vi "test_sicm_main2.vi"() -> ()   [LabVIEW 2016]
uses:
  <vilib>/rvi/DesktopExecutionNode/Execution/niFpgaDEN_Execute.vi
  <vilib>/rvi/DesktopExecutionNode/DesktopExecutionNode.xnode
panel:
  out "Baseline":dbl[](graph)
  out "Height":dbl[](graph)
  out "current":dbl[](graph)
  out "Baseline":T1(array[cluster])
  out "Debug":T2(array[cluster])
  out "Trigger":T3(array[cluster])
  in  "sicm.p.modes":T4
  in  "sicm.display":cluster{"sicm.ptsAfterTrig":u16}={"sicm.ptsAfterTrig"=10}
  in  "sicm.p.params":T5={"sicm.p.setPoint"=0.9700002670288086, "sicm.p.setPointFrac"=-33.328125, "stepDown"=0.001999974250793457, "retractHeight"=-0.19999998807907104, "adaptiveMin"=0.099609375}
  out "heightOut":T6(array[cluster])
  in  "enablethicks":i32=2000
  out "Progress":dbl(slide)=0.9999 scale=0.0..1.0
  in  "sicm.i.current":T7
  in  "sicm.p.clocks":T8={"inverseDecimation"=0.03332996368408203, "decimation"=10, "waveSize"=128, "pixelDecimation"=0}
  in  "sicm.blc.p.params":T9={"se.blc.p.postRetractDelay"=1000, "se.blc.p.windowSize"=20, "se.blc.p.updateFactor"=-5, "blc.resetBackground"=FALSE}
  in  "d0":dbl=0.3
  in  "D":dbl=0.05
  in  "Idc":dbl=5000.0
  in  "Simulation ticks":i32=10000
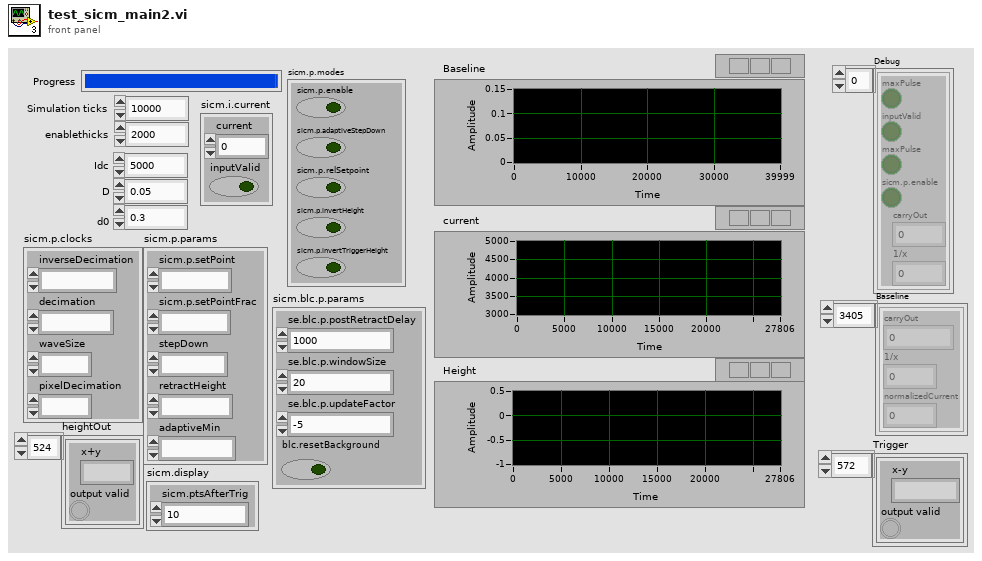
[diagram p1: front panel]
types:
  T1 = cluster{"carryOut":fxp<+/-,22,2>, "1/x":fxp<+/-,32,24>, "normalizedCurrent":fxp<+,20,1>}[]
  T2 = cluster{"maxPulse":bool, "inputValid":bool, "maxPulse":bool, "sicm.p.enable":bool, "carryOut":fxp<+/-,22,2>, "1/x":fxp<+/-,27,24>}[]
  T3 = cluster{"x-y":fxp<+/-,22,4>, "output valid":bool}[]
  T4 = cluster{"sicm.p.enable":bool, "sicm.p.adaptiveStepDown":bool, "sicm.p.relSetpoint":bool, "sicm.p.invertHeight":bool, "sicm.p.invertTriggerHeight":bool}
  T5 = cluster{"sicm.p.setPoint":fxp<+,20,0>, "sicm.p.setPointFrac":fxp<+/-,20,14>, "stepDown":fxp<+/-,28,4>, "retractHeight":fxp<+/-,28,4>, "adaptiveMin":fxp<+,10,0>}
  T6 = cluster{"x+y":fxp<+/-,28,2>, "output valid":bool}[]
  T7 = cluster{"current":fxp<+/-,24,16>, "inputValid":bool}
  T8 = cluster{"inverseDecimation":fxp<+,22,0>, "decimation":u16, "waveSize":u16, "pixelDecimation":u16}
  T9 = cluster{"se.blc.p.postRetractDelay":u16, "se.blc.p.windowSize":u16, "se.blc.p.updateFactor":i16, "blc.resetBackground":bool}
  T10 = cluster{"x-y":fxp<+/-,22,4>, "output valid":bool}
  T11 = cluster{"x+y":fxp<+/-,28,2>, "output valid":bool}
  T12 = cluster{"maxPulse":bool, "inputValid":bool, "maxPulse":bool, "sicm.p.enable":bool, "carryOut":fxp<+/-,22,2>, "1/x":fxp<+/-,27,24>}
  T13 = cluster{"carryOut":fxp<+/-,22,2>, "1/x":fxp<+/-,32,24>, "normalizedCurrent":fxp<+,20,1>}
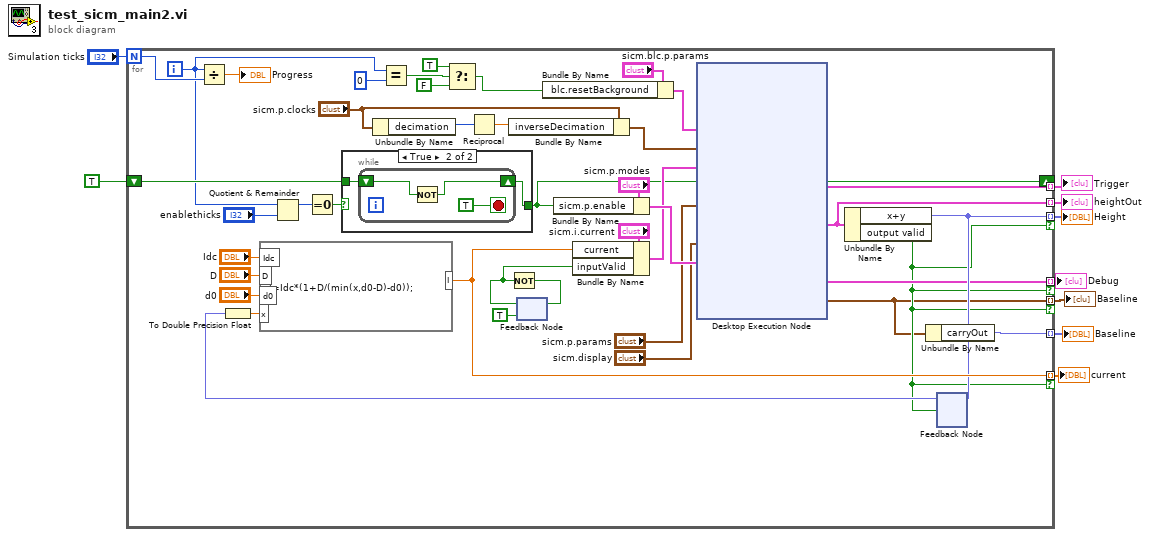
[diagram p0: block diagram]
diagram:
  n1 = for {
    N: "Simulation ticks" -> [w48]
    tunnel: [w35] -> w8 mode=indexing if=w21
    tunnel: [w34] -> w7 mode=indexing
    tunnel: [w31] -> w6 mode=indexing
    tunnel: [w28] -> w5 mode=indexing if=w21
    shift-right: [w20] -> _
    shift-left: TRUE -> [w23]
    tunnel: [w22] -> w3 mode=indexing if=w21
    tunnel: [w19] -> w2 mode=indexing if=w21
    tunnel: [w18] -> w1 mode=indexing
    i -> [w15]
    n2 = Divide(x=w15, y=w48) -> (x/y=→"Progress":dbl)
    n3 = Quotient & Remainder(x=w15, y="enablethicks") -> (x-y*floor(x/y)=w25:i32)  [unwired: 1 out]
    n4 = Equal To 0?(x=w25) -> (x = 0?=w24:bool)
    n5 = case shown="True" w24 {
      tunnel: w23 -> [w51 w53]
      tunnel: [w51 w52] -> w20
      frame False {
      }
      frame True {
        n6 = while {
          shift-right: [w55] -> w52
          shift-left: w53 -> [w54]
          stop <- TRUE stop-if-true
          n7 = Not(x=w54) -> (.not. x?=w55:bool)
        }
      }
    }
    n8 = Unbundle By Name("sicm.p.clocks") -> ("decimation"=w36:u16)
    n9 = Equal?(x=w15, y=0) -> (x = y?=w12:bool)
    n10 = Select(t=TRUE, s=w12, f=FALSE) -> (s? t:f=w13:bool)
    n11 = Reciprocal(x=w36) -> (1/x=w37:dbl)
    n12 = Bundle By Name(cluster="sicm.p.clocks", "inverseDecimation"=w37) -> (w39:T8)
    n13 = feedback #1(TRUE) -> (w40:bool)
    n14 = Not(x=w40) -> (.not. x?=w42:bool)
    n15 = feedback-in #1(w42) -> ()
    n16 = Bundle By Name(cluster="sicm.blc.p.params", "blc.resetBackground"=w13) -> (w16:T9)
    n17 = Bundle By Name(cluster="sicm.p.modes", "sicm.p.enable"=w20) -> (w50:T4)
    n18 = feedback #2() -> (w30:fxp<+/-,28,2>)  [unwired: 1 in]
    n19 = To Double Precision Float(number=w30) -> (double precision float=w44:dbl)
    n20 = formula code="I=Idc*(1+D/(min(x,d0-D)-d0));"("Idc"="Idc", "D"="D", "d0"="d0", "x"=w44) -> ("I"=w35:dbl)
    n21 = Bundle By Name(cluster="sicm.i.current", "current"=w35, "inputValid"=w40) -> (w43:T7)
    n22 = xnode "Desktop Execution Node"("sicm.blc.p.params"=w16, "sicm.p.clocks"=w39, "sicm.i.current"=w43, "sicm.p.params"="sicm.p.params", "sicm.display"="sicm.display", "sicm.p.modes"=w50) -> ("sicm.triggerHeight"=w34:T10, "heightOut"=w31:T11, "debug"=w22:T12, "sicm.Baseline"=w19:T13)  [unwired: 1 in, 1 out]
    n23 = Unbundle By Name(w31) -> ("x+y"=w28:fxp<+/-,28,2>, "output valid"=w21:bool)
    n24 = Unbundle By Name(w19) -> ("carryOut"=w18:fxp<+/-,22,2>)
    n25 = feedback-in #2(w28, w21) -> ()
  }
  "current" <- w8
  "Trigger" <- w7
  "heightOut" <- w6
  "Height" <- w5
  "Debug" <- w3
  "Baseline" <- w2
  "Baseline" <- w1
